vi "String.Convert CSV Line with Quotes to 1D Array.vi"(8 "error in":errorcluster, 11 "CSV String":string) -> (0 "error out":errorcluster, 3 "Array":string[](array[string]))   [LabVIEW 2024, in "EQMF.lvlib" / "String Utils.lvlib"]
uses:
  String Utils.lvlib
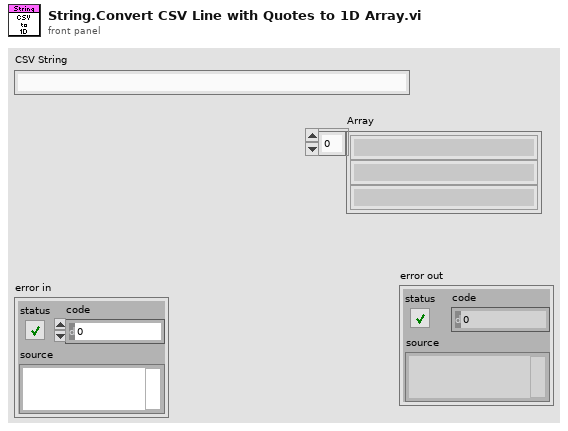
[diagram p1: front panel]
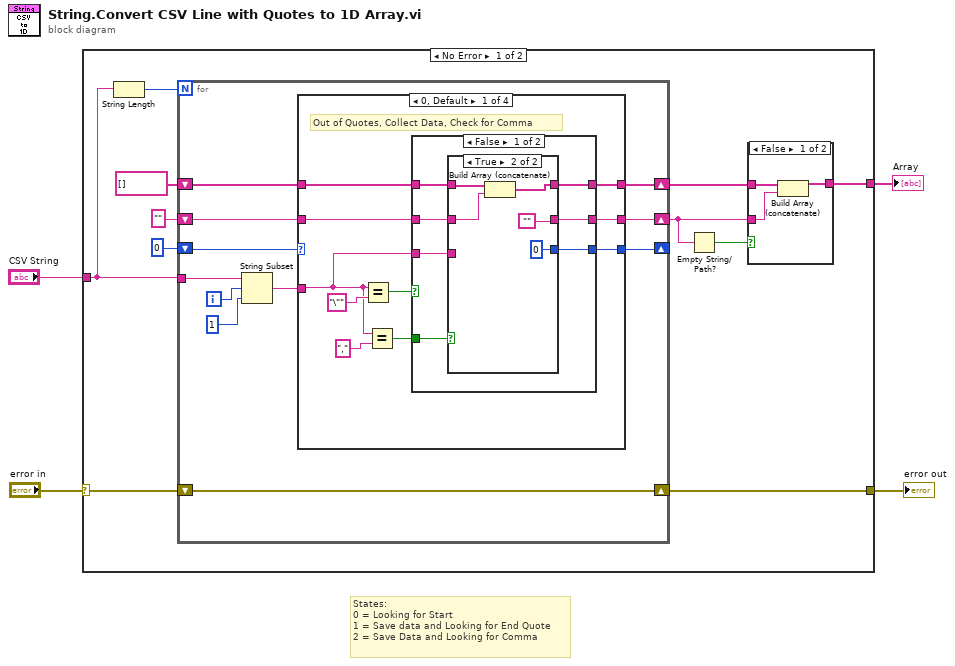
[diagram p0: block diagram]
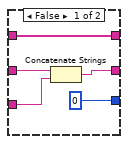
[diagram p3: hidden frame]
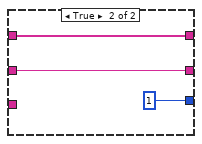
[diagram p4: hidden frame]
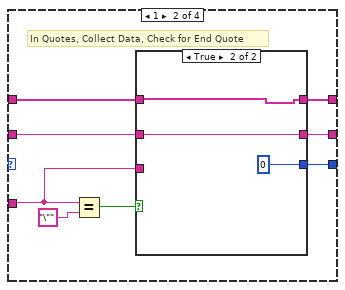
[diagram p5: hidden frame]
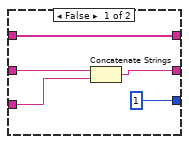
[diagram p6: hidden frame]
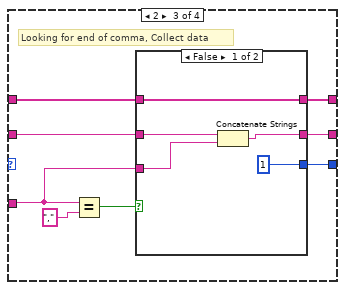
[diagram p7: hidden frame]
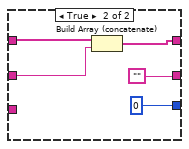
[diagram p8: hidden frame]
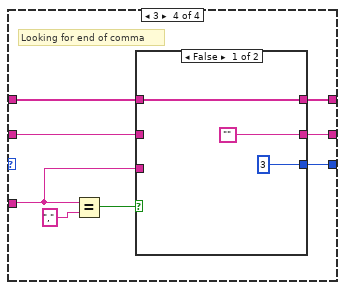
[diagram p9: hidden frame]
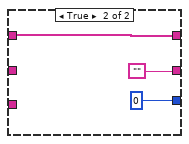
[diagram p10: hidden frame]
diagram:
  # "States:\n0 = Looking for Start\n1 = Save data and Looking for End Quote\n2 = Save Data and Looking for Comma"
  n1 = case shown="No Error" "error in" {
    selector: "error in" -> [w15 w109]
    tunnel: [w14 w109] -> w3
    tunnel: "CSV String" -> [w12 _]
    tunnel: [w8 _] -> w1
    frame No Error {
      n2 = String Length(string=w12) -> (length=w9:i32)
      n3 = for {
        N: w9 -> [_]
        shift-right: [w30] -> w14
        shift-left: w15 -> [w30]
        shift-right: [w21] -> w7
        shift-left: string[] [] -> [w22]
        shift-right: [w23] -> w6
        shift-left: "" -> [w24]
        shift-right: [w25] -> _
        shift-left: 0 -> [w26]
        tunnel: w12 -> [w29]
        i -> [w28]
        n4 = String Subset(string=w29, offset (0)=w28, length (rest)=1 ("length (rest)")) -> (substring=w27:string)
        n5 = case shown="0, Default" w26 {
          tunnel: w27 -> [w32 w61 w77 w95]
          tunnel: [w39 w66 w82 w100] -> w25
          tunnel: w24 -> [w38 w65 w81 w99]
          tunnel: [w37 w64 w80 w98] -> w23
          tunnel: w22 -> [w36 w63 w79 w97]
          tunnel: [w35 w62 w78 w96] -> w21
          frame 0, Default {
            # "Out of Quotes, Collect Data, Check for Comma"
            n6 = Equal?(x=w32, y="\"") -> (x = y?=w34:bool)
            n7 = Equal?(x=w32, y=",") -> (x = y?=w31:bool)
            n8 = case shown="False" w34 {
              tunnel: [w44 1] -> w39
              tunnel: w38 -> [w47 w58]
              tunnel: [w46 w58] -> w37
              tunnel: w36 -> [w43 w59]
              tunnel: [w42 w59] -> w35
              tunnel: w32 -> [w45 _]
              tunnel: w31 -> [w41 _]
              frame False {
                n9 = case shown="True" w41 {
                  tunnel: w47 -> [w52 w53]
                  tunnel: [w51 ""] -> w46
                  tunnel: w45 -> [w50 _]
                  tunnel: [0 0] -> w44
                  tunnel: w43 -> [w48 w55]
                  tunnel: [w48 w54] -> w42
                  frame False {
                    n10 = Concatenate Strings(w52, w50) -> (w51:string)
                  }
                  frame True {
                    n11 = Build Array (concatenate)(w55, w53) -> (w54:string[])
                  }
                }
              }
              frame True {
              }
            }
          }
          frame 1 {
            # "In Quotes, Collect Data, Check for End Quote"
            n12 = Equal?(x=w61, y="\"") -> (x = y?=w67:bool)
            n13 = case shown="True" w67 {
              tunnel: [1 0] -> w66
              tunnel: w65 -> [w73 w74]
              tunnel: [w72 w74] -> w64
              tunnel: w63 -> [w70 w75]
              tunnel: [w70 w75] -> w62
              tunnel: w61 -> [w71 _]
              frame False {
                n14 = Concatenate Strings(w73, w71) -> (w72:string)
              }
              frame True {
              }
            }
          }
          frame 2 {
            # "Looking for end of comma, Collect data"
            n15 = Equal?(x=w77, y=",") -> (x = y?=w83:bool)
            n16 = case shown="False" w83 {
              tunnel: [1 0] -> w82
              tunnel: w81 -> [w89 w91]
              tunnel: [w88 ""] -> w80
              tunnel: w79 -> [w86 w93]
              tunnel: [w86 w92] -> w78
              tunnel: w77 -> [w87 _]
              frame False {
                n17 = Concatenate Strings(w89, w87) -> (w88:string)
              }
              frame True {
                n18 = Build Array (concatenate)(w93, w91) -> (w92:string[])
              }
            }
          }
          frame 3 {
            # "Looking for end of comma"
            n19 = Equal?(x=w95, y=",") -> (x = y?=w101:bool)
            n20 = case shown="False" w101 {
              tunnel: [3 0] -> w100
              tunnel: w99 -> [_ _]
              tunnel: ["" ""] -> w98
              tunnel: w97 -> [w105 w106]
              tunnel: [w105 w106] -> w96
              tunnel: w95 -> [_ _]
              frame False {
              }
              frame True {
              }
            }
          }
        }
      }
      n21 = Empty String/Path?(string/path=w6) -> (empty?=w5:bool)
      n22 = case shown="False" w5 {
        tunnel: [w18 w19] -> w8
        tunnel: w7 -> [w17 w19]
        tunnel: w6 -> [w16 _]
        frame False {
          n23 = Build Array (concatenate)(w17, w16) -> (w18:string[])
        }
        frame True {
        }
      }
    }
    frame Error {
    }
  }
  "Array" <- w1
  "error out" <- w3
